vi "NewFlexUIActorVIs.vi"(8 "error in (no error)":errorcluster, 11 "FlexUIActorMaker in":refnum<class "FlexUIActorMaker.lvclass">) -> (0 "error out":errorcluster, 3 "FlexUIActorMaker out":refnum<class "FlexUIActorMaker.lvclass">)   [LabVIEW 2016, in "FlexUIActorMaker.lvlib" / "FlexUIActorMaker.lvclass"]
uses:
  FlexUIActorMaker.lvclass
  FlexUIActorMaker.lvclass/FlexUIActorMaker.ctl
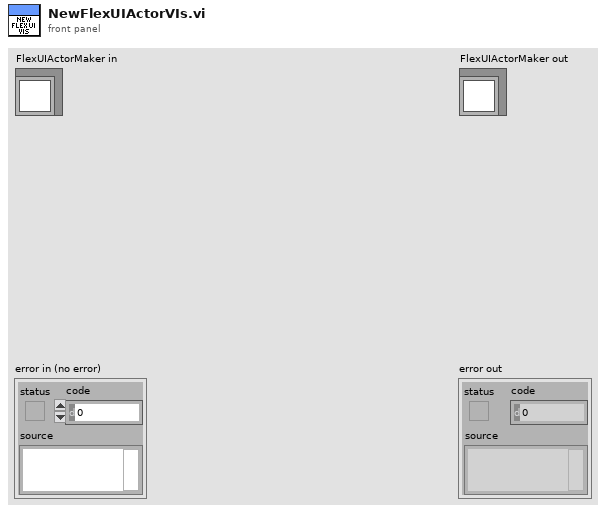
[diagram p1: front panel]
types:
  T1 = enum32{"invalid scope", "public", "private", "protected", "community"}
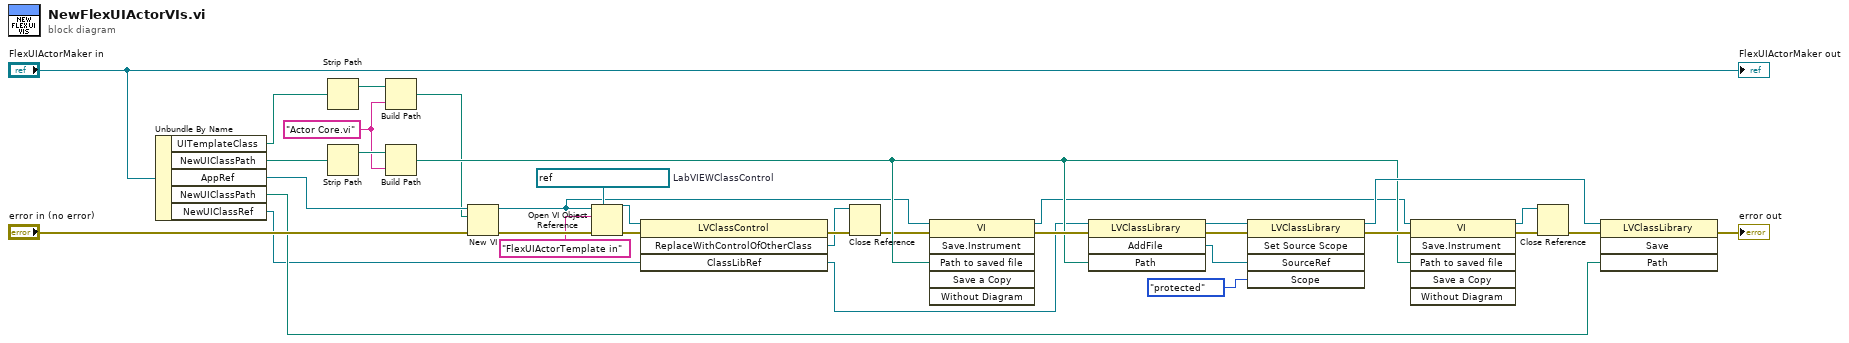
[diagram p0: block diagram]
diagram:
  w21 = refnum<vi> refnum  # LabVIEWClassControl
  w28 = "Actor Core.vi" ("name or relative path")
  n1 = Unbundle By Name("FlexUIActorMaker in") -> ("UITemplateClass"=w12:path, "NewUIClassPath"=w30:path, "AppRef"=w33:refnum<vi>, "NewUIClassPath"=w27:path, "NewUIClassRef"=w4:refnum<vi>)
  n2 = Strip Path(path=w12) -> (stripped path=w31:path)  [unwired: 1 out]
  n3 = Strip Path(path=w30) -> (stripped path=w29:path)  [unwired: 1 out]
  n4 = Build Path(base path=w31, name or relative path=w28) -> (appended path=w8:path)
  n5 = Build Path(base path=w29, name or relative path=w28) -> (appended path=w9:path)
  n6 = New VI(8:"error in (no error)", 10:w8, 11:w33) -> (0:w25:errorcluster, 3:w2:refnum<vi>)  [unwired: 4 in]
  n7 = Open VI Object Reference(7:w21, 8:w25, 10:"FlexUIActorTemplate in" ("Control Name"), 11:w2) -> (0:w23:errorcluster, 3:w22:refnum<vi>)
  n8 = invoke class="LVClassControl" method="ReplaceWithControlOfOtherClass"(reference=w22, error in=w23, "ClassLibRef"=w4) -> (error out=w11:errorcluster, "ReplaceWithControlOfOtherClass"=w5:refnum<vi>, "ClassLibRef"=w3:refnum<vi>)  [unwired: 1 in, 1 out]
  n9 = Close Reference(reference=w5, error in (no error)=w11) -> (error out=w6:errorcluster)
  n10 = invoke class="VI" method="Save.Instrument"(reference=w2, error in=w6, "Path to saved file"=w9) -> (reference out=w1:refnum<vi>, error out=w10:errorcluster)  [unwired: 3 in, 4 out]
  n11 = invoke class="LVClassLibrary" method="AddFile"(reference=w3, error in=w10, "Path"=w9) -> (reference out=w18:refnum<vi>, error out=w19:errorcluster, "AddFile"=w17:refnum<vi>)  [unwired: 1 in, 1 out]
  n12 = invoke class="LVClassLibrary" method="Set Source Scope"(reference=w18, error in=w19, "SourceRef"=w17, "Scope"=T1."protected" ("scope")) -> (reference out=w15:refnum<vi>, error out=w16:errorcluster)  [unwired: 1 in, 3 out]
  n13 = invoke class="VI" method="Save.Instrument"(reference=w1, error in=w16, "Path to saved file"=w9) -> (reference out=w13:refnum<vi>, error out=w7:errorcluster)  [unwired: 3 in, 4 out]
  n14 = Close Reference(reference=w13, error in (no error)=w7) -> (error out=w14:errorcluster)
  n15 = invoke class="LVClassLibrary" method="Save"(reference=w15, error in=w14, "Path"=w27) -> (error out=→"error out":errorcluster)  [unwired: 1 in, 3 out]
  "FlexUIActorMaker out" <- "FlexUIActorMaker in"
